vi "posicionador3_2_8_ElBueno_4.vi"() -> ()   [LabVIEW 2015]
uses:
  <vilib>/Instr/_visa.llb/VISA Configure Serial Port (Instr).vi
panel:
  out "Caracterización Terminada":bool
  in  "Puerto Serial del Gaussmetro":refnum<visa-resource-name>="COM5"
  in  "Ruta de archivo de medición":path=path "C:/Users/PIV/Desktop/Enrico/prueba1.txt"
  in  "Dato de entrada para\nobtención de flujo magnético 2":string=":MEASure:FLUX?\n"
  out "Medición de campo magnético \nen Teslas [T]":string
  out "?":string="mm"
  out "?":string="mm"
  in  "Listo Y":bool
  in  "Listo X":bool
  in  "Abajo":bool
  in  "Arriba":bool
  in  "Derecha":bool
  in  "Izquierda":bool
  out "Posiciòn en eje X":i32
  out "Posiciòn en eje Y":i32
  in  "Longitud del imán":i32
  in  "Altura del imán":i32
  in  "Puerto Serial de Arduino":refnum<visa-resource-name>="COM12"
  # "Manual de uso para sistema de monitoreo y control de lecturas de flujo magnético y desplazamiento de posicionador:\n\nSECCI`ÓN DE IDE DE ARDUINO: El archivo se encuentra bajo la x\n\n1.  Los pines para la conexión del driver del motor con el arduino están indicados en el archivo \"motor2.ino\" mediante las variables \"DirPin\", \"StepPin\", \"EnnablePin\" para el motor en X, y \"DirPin2\", \"StepPin2\", \"EnnablePin2\", para el motor en Y. El primer pin refiere a la Dirección; el segundo es el pin para mandarle el tren de pulsos y el tercero para habilitar el motor.\n2.  Para modificar el desplazamiento de 1mm de ambos motores, se deberá modificar el archivo \"motor2.ino\" en la sección después del loop denominada \"void stepMotor\" y \"void Stepmotor2, modificar la variable steps por la cantidad de desplazamiento deseado, tomando en cuenta que steps = 1000 = 1mm de desplazamiento.\n3.  En el apartado \"Puerto Serial de Arduino\" en la parte superior izquierda, indicar el puerto serial del Arduino. Para verificar en què puerto se localiza, dirigirse al menù inicio y escribir \"Administrador de dispositivos\". Seguido de esto se darà click en la opciòn con el mismo nombre y, en la ventaja que emerge, se buscarà el apartado \"Puertos COM y LPT\". El puerto del Arduino lleva por nombre inicial \"Arduino\".\n4.  Para seleccionar el puerto del Gaussmetro, dirigirse como en el paso anterior al Administrador de dispositivos y en el apartado Puerto COM y LPT buscar el nombre \"Prolific USB-to-Serial Comm Port\", y el nombre del puerto se especificarà entre parèntesis. Este nombre de puerto se especificará en el apartado \"Puerto Serial del Gaussmetro\" ubicado debajo del apartado \"Puerto Serial de Arduino\". \n5.  Ingresar la longitud [en mm] del imán.\n6.  Ingresar el alto [en mm] del imán\n7.  Crear un archivo de texto .txt en la computadora (ubicación a elección) para guardar archivos \n8.  En el apartado \"Ruta de archivo de medición\" se deberá introducir la ubicación del archivo creado en el paso anterior. De esta manera, se introducirán las mediciones en este archivo.\n9.  En el apartado \"Dato de entrada para obtención de campo magnético\" se encuentra escrito el comando paara que el Gaussmetro arroje la medición de campo magnético.\n10.  Colocar el imán a caracterizar de forma que la probeta se encuentre del lado superior izquierdo de este. Esto debido a que el movimiento horizontal es hacia la derecha, y el movimiento vertical es hacia abajo.\n11.  Iniciar programa mediante la flecha (con dirección a la derecha) blanca en la parte superior izquierda del panel frontal o Ctrl+R.\n12. Verificar Conexión entre el Arduino y el posicionador. Esto se realiza observando un foco led color naranja en el motor (esto indica que la comunicación serial fue exitosa).\n13.  En caso de estar apagada la luz led naranja del motor, se deberá reiniciar el programa. Esto se consigue oprimiendo el boton \"Listo X\". Al hacer esto, se encenderá el led naranja, y de esta manera se procede a apagar el programa mediante el botón rojo de la parte superior izquierda del panel frontal. Después de realizar esta acciòn, volver a ejecutar el progama oprimiendo la flecha blanca a la izquierda del botón rojo o CTRL+R\n14.  Se deberá iniciar colocando la posición inicial en X (Derecha e Izquierda). Una vez finalizada la posición inicial en X, oprimir el botón \"Listo X\". Al finalizar, deberá parpadear una vez el foco led naranja y se volverá a encender.\n15.  Seguido, se colocará la  posición inicial en Y (Arriba y Abajo). Una vez finalizada la posición inicial en Y, oprimir el botón \"Listo Y\". Al finalizar, deberá parpadear una vez el foco led naranja y se volverá a encender.\n16.  Se comenzará la caracterización deseada.\n\n\nCreado por:\nSebastian A. Reyes Romero\nContacto: rerosa@ier.unam.mx"
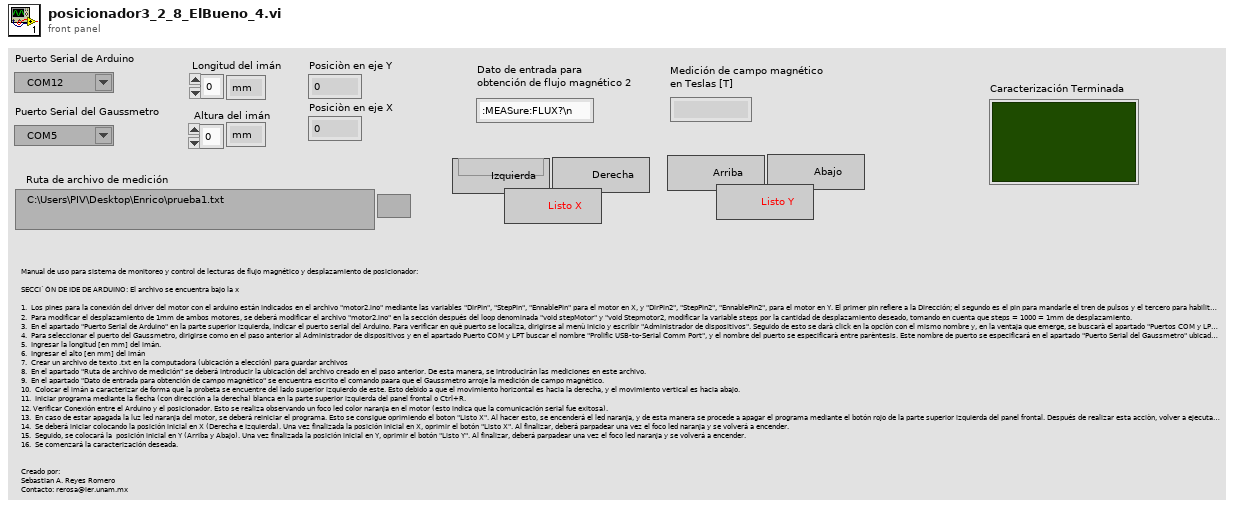
[diagram p1: front panel]
types:
  T1 = enum16{"open", "open or create", "create or replace", "create", "open (read only)"}
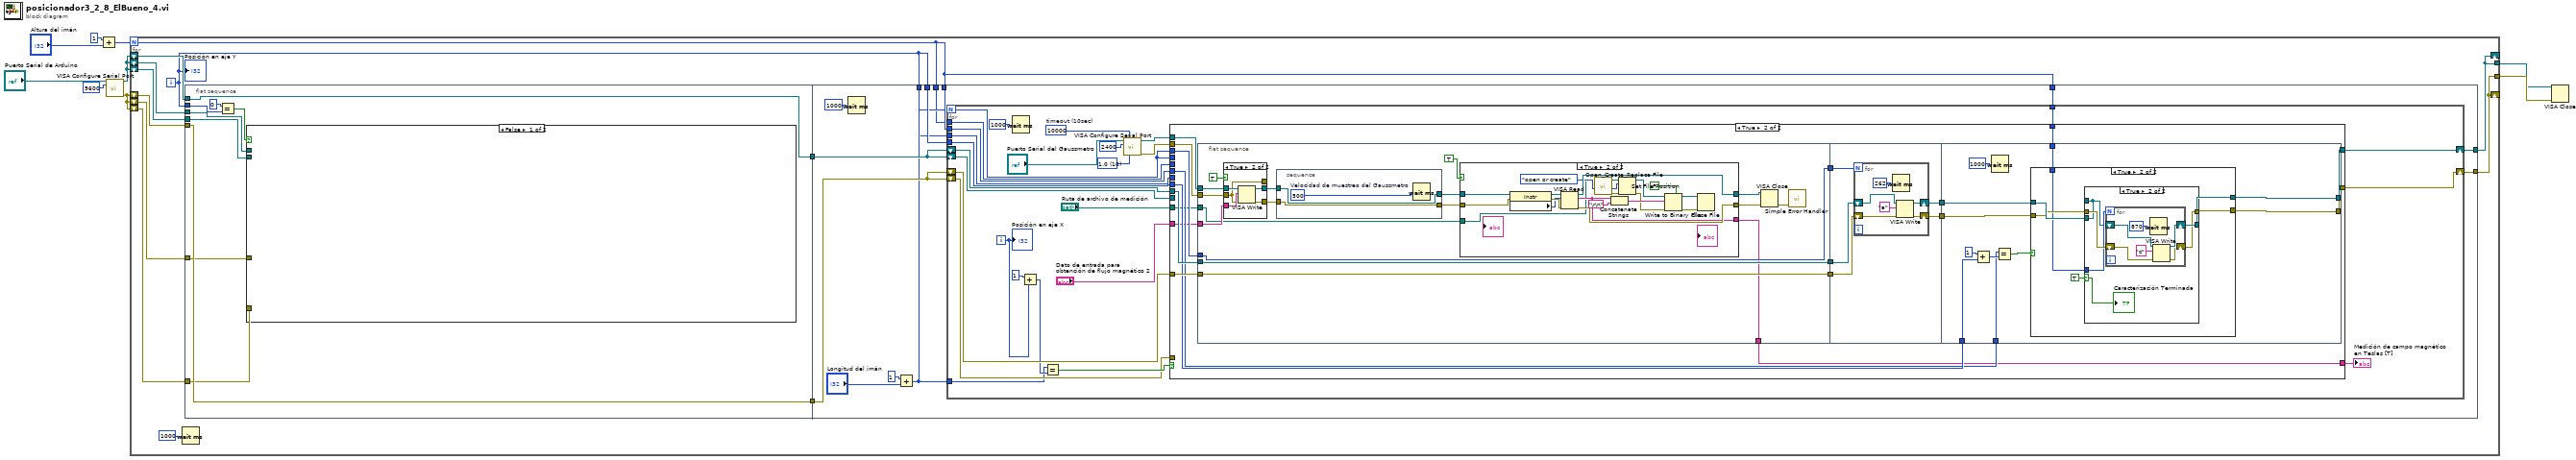
[diagram p0: block diagram]
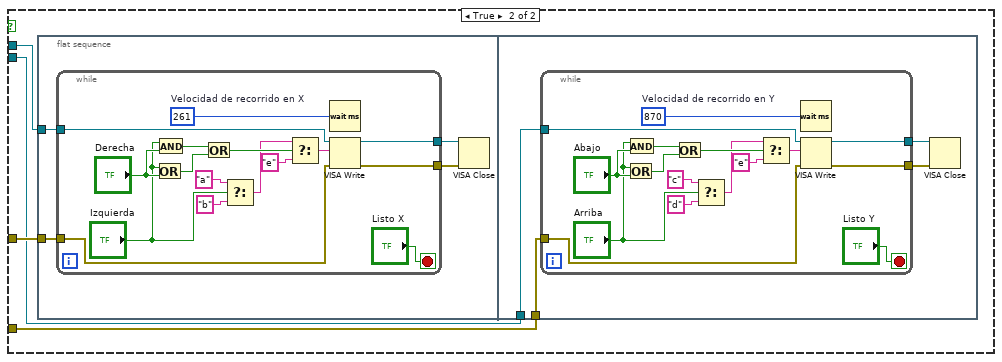
[diagram p2: hidden frame]
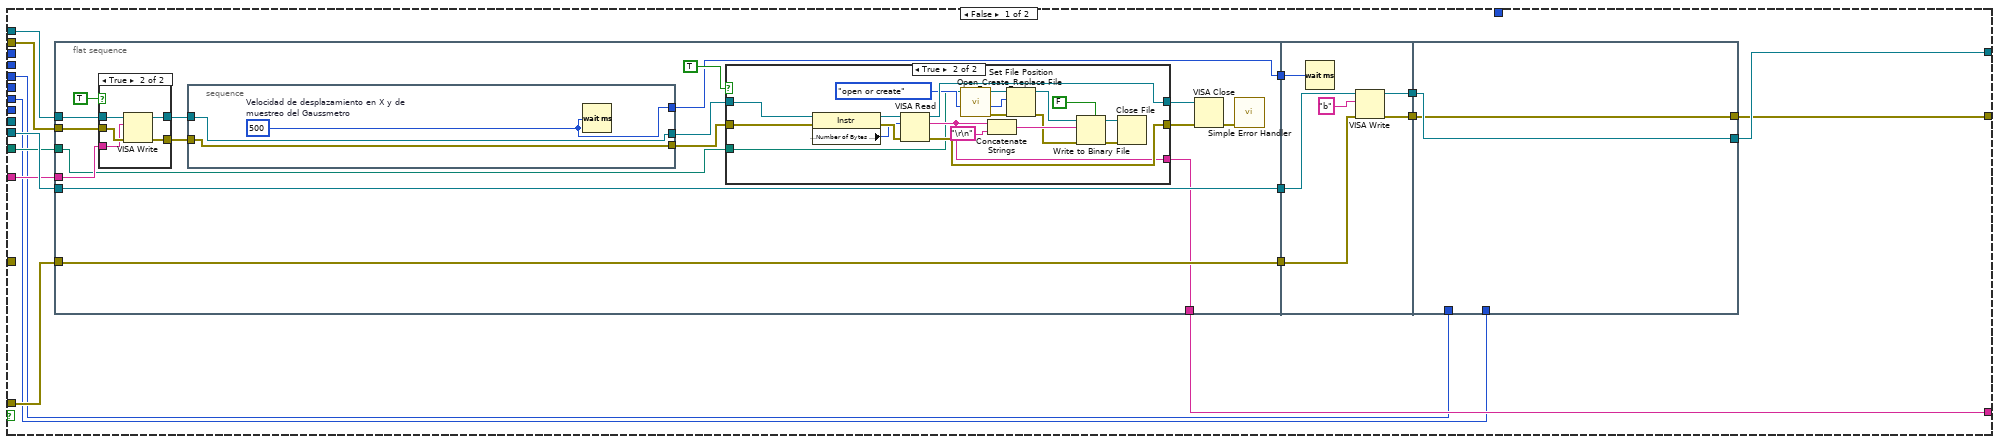
[diagram p3: hidden frame]
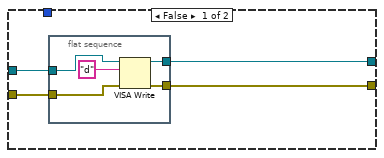
[diagram p8: hidden frame]
diagram:
  n1 = Add(x=1, y="Altura del imán") -> (x+y=w5:i32)
  n2 = call-poly "VISA Configure Serial Port"("VISA resource name"="Puerto Serial de Arduino", "baud rate (9600)"=u32 9600) -> ("VISA resource name out"=w3:refnum<visa-resource-name>, "error out"=w4:errorcluster)  [unwired: 12 in]
  n3 = for {
    N: w5 -> [w10]
    shift-right: [w12] -> _
    shift-right: [w13] -> _
    shift-left: w4 -> [w22]
    shift-left: w3 -> [w18]
    shift-left: w4 -> [w17]
    shift-left: w4 -> [w16]
    shift-left: w3 -> [w14]
    shift-left: w3 -> [w15]
    tunnel: [w13] -> w2
    tunnel: [w12] -> w1
    i -> [w11]
    n4 = Wait (ms)(milliseconds to wait=u32 1000) -> ()  [unwired: 1 out]
    n5 = flat-sequence {
      tunnel: w22 -> [w31]
      tunnel: [w28] -> w20
      tunnel: [w31] -> w19
      tunnel: w18 -> [w27]
      tunnel: w17 -> [w30]
      tunnel: w16 -> [w29]
      tunnel: w15 -> [w28]
      tunnel: w14 -> [w26]
      tunnel: w11 -> [w25]
      tunnel: [w87] -> w13
      tunnel: [w88] -> w12
      tunnel: w11 -> [w84]
      tunnel: w10 -> [w83]
      tunnel: w20 -> [w86]
      tunnel: w19 -> [w85]
      tunnel: w10 -> [w78]
      tunnel: w11 -> [w77]
      tunnel: w10 -> [w76]
      frame #0 {
        n6 = Equal?(x=0, y=w25) -> (x = y?=w23:bool)
        n7 = case shown="False" w23 {
          tunnel: w30 -> [_ w35]
          tunnel: w29 -> [_ w34]
          tunnel: w27 -> [_ w33]
          tunnel: w26 -> [_ w32]
          frame False {
          }
          frame True {
            n8 = flat-sequence {
              tunnel: w32 -> [w39]
              tunnel: w35 -> [w38]
              tunnel: w33 -> [w59]
              tunnel: w34 -> [w58]
              frame #0 {
                n9 = while {
                  tunnel: w39 -> [w46]
                  tunnel: w38 -> [w45]
                  tunnel: [w41] -> w37
                  tunnel: [w40] -> w36
                  stop <- "Listo X" stop-if-true
                  w42 = u32 261  # Velocidad de recorrido en X
                  n10 = Or(x="Izquierda", y="Derecha") -> (x .or. y?=w52:bool)
                  n11 = And(x="Izquierda", y="Derecha") -> (x .and. y?=w54:bool)
                  n12 = Or(x=w54, y=w52) -> (x .or. y?=w51:bool)
                  n13 = Select(t="a", s="Izquierda", f="b") -> (s? t:f=w44:string)
                  n14 = Select(t=w44, s=w51, f="e") -> (s? t:f=w47:string)
                  n15 = Wait (ms)(milliseconds to wait=w42) -> ()  [unwired: 1 out]
                  n16 = VISA Write(VISA resource name=w46, write buffer=w47, error in (no error)=w45) -> (VISA resource name out=w40:refnum<visa-resource-name>, error out=w41:errorcluster)  [unwired: 1 out]
                }
                n17 = VISA Close(VISA resource name=w36, error in (no error)=w37) -> ()  [unwired: 1 out]
              }
              frame #1 {
                n18 = while {
                  tunnel: w59 -> [w66]
                  tunnel: w58 -> [w65]
                  tunnel: [w61] -> w57
                  tunnel: [w60] -> w56
                  stop <- "Listo Y" stop-if-true
                  w62 = u32 870  # Velocidad de recorrido en Y
                  n19 = Or(x="Arriba", y="Abajo") -> (x .or. y?=w73:bool)
                  n20 = And(x="Arriba", y="Abajo") -> (x .and. y?=w74:bool)
                  n21 = Or(x=w74, y=w73) -> (x .or. y?=w72:bool)
                  n22 = Select(t="c", s="Arriba", f="d") -> (s? t:f=w63:string)
                  n23 = Select(t=w63, s=w72, f="e") -> (s? t:f=w67:string)
                  n24 = Wait (ms)(milliseconds to wait=w62) -> ()  [unwired: 1 out]
                  n25 = VISA Write(VISA resource name=w66, write buffer=w67, error in (no error)=w65) -> (VISA resource name out=w60:refnum<visa-resource-name>, error out=w61:errorcluster)  [unwired: 1 out]
                }
                n26 = VISA Close(VISA resource name=w56, error in (no error)=w57) -> ()  [unwired: 1 out]
              }
            }
          }
        }
      }
      frame #1 {
        n27 = Wait (ms)(milliseconds to wait=u32 1000) -> ()  [unwired: 1 out]
        n28 = Add(x=1, y="Longitud del imán") -> (x+y=w80:i32)
        n29 = for {
          N: w80 -> [w109]
          shift-right: [w112] -> w88
          shift-left: w86 -> [w114]
          shift-right: [w111] -> w87
          shift-left: w85 -> [w113]
          shift-left: w86 -> [w110]
          shift-left: w85 -> [w108]
          tunnel: w80 -> [w104]
          tunnel: w84 -> [w103]
          tunnel: w83 -> [w102]
          tunnel: w78 -> [w91]
          tunnel: w77 -> [w90]
          tunnel: w76 -> [w89]
          i -> [w107]
          w94 = u16 10 items=["1.0"=10, "1.5"=15, "2.0"=20] ("stop bits (10: 1 bit)")
          w97 = u32 10000  # timeout (10sec)
          n30 = Wait (ms)(milliseconds to wait=u32 1000) -> ()  [unwired: 1 out]
          n31 = Add(x=1, y=w107) -> (x+y=w105:i32)
          n32 = Equal?(x=w104, y=w105) -> (x = y?=w115:bool)
          n33 = call-poly "VISA Configure Serial Port"("VISA resource name"="Puerto Serial del Gaussmetro", "timeout (10sec)"=w97, "baud rate (9600)"=u32 2400, "stop bits (10: 1 bit)"=w94) -> ("VISA resource name out"=w93:refnum<visa-resource-name>, "error out"=w92:errorcluster)  [unwired: 5 in, 5 out]
          n34 = case shown="True" w115 {
            tunnel: w114 -> [_ w206]
            tunnel: w113 -> [_ w205]
            tunnel: [w129 w204] -> w112
            tunnel: [w128 w203] -> w111
            tunnel: w109 -> [_ w202]
            tunnel: w110 -> [w131 _]
            tunnel: w108 -> [w130 _]
            tunnel: w109 -> [_ _]
            tunnel: w103 -> [_ w199]
            tunnel: w102 -> [_ w198]
            tunnel: [w124 w194] -> w100
            tunnel: "Dato de entrada para\nobtención de flujo magnético 2" -> [w123 w193]
            tunnel: "Ruta de archivo de medición" -> [w122 w192]
            tunnel: w93 -> [w121 w191]
            tunnel: w92 -> [w120 w190]
            tunnel: w91 -> [w117 _]
            tunnel: w90 -> [w116 _]
            tunnel: w89 -> [_ w189]
            frame False {
              n35 = flat-sequence {
                tunnel: w130 -> [w147]
                tunnel: w131 -> [w148]
                tunnel: [w148] -> w127
                tunnel: [w147] -> w126
                tunnel: [w137] -> w125
                tunnel: [w136] -> w124
                tunnel: w123 -> [w135]
                tunnel: w122 -> [w134]
                tunnel: w121 -> [w133]
                tunnel: w120 -> [w132]
                tunnel: w127 -> [w186]
                tunnel: w126 -> [w185]
                tunnel: w125 -> [w181]
                tunnel: [w184] -> w119
                tunnel: [w183] -> w118
                tunnel: [w187] -> w128
                tunnel: [w188] -> w129
                tunnel: w119 -> [w188]
                tunnel: w118 -> [w187]
                tunnel: w117 -> [_]
                tunnel: w116 -> [_]
                frame #0 {
                  n36 = case shown="True" TRUE ("write") {
                    tunnel: [w153 w158] -> w141
                    tunnel: w133 -> [w152 w157]
                    tunnel: w132 -> [w153 w156]
                    tunnel: [w152 w155] -> w139
                    tunnel: w135 -> [_ w154]
                    frame False {
                    }
                    frame True {
                      n37 = VISA Write(VISA resource name=w157, write buffer=w154, error in (no error)=w156) -> (VISA resource name out=w155:refnum<visa-resource-name>, error out=w158:errorcluster)  [unwired: 1 out]
                    }
                  }
                  n38 = stacked-sequence {
                    tunnel: w141 -> [w151]
                    tunnel: [w151] -> w140
                    tunnel: w139 -> [w150]
                    tunnel: [w150] -> w138
                    tunnel: [w149] -> w137
                    frame #0 {
                      w149 = u32 500  # Velocidad de desplazamiento en X y de muestreo del Gaussmetro
                      n39 = Wait (ms)(milliseconds to wait=w149) -> ()  [unwired: 1 out]
                    }
                  }
                  n40 = case shown="True" TRUE ("read") {
                    tunnel: w140 -> [w160 w177]
                    tunnel: [w160 w174] -> w145
                    tunnel: [w159 w180] -> w144
                    tunnel: w138 -> [w159 w179]
                    tunnel: [_ w162] -> w136
                    tunnel: w134 -> [_ w161]
                    frame False {
                    }
                    frame True {
                      n41 = property class="Instr"(reference=w179, error in=w177) -> (reference out=w178:refnum<visa-resource-name>, error out=w176:errorcluster, "Serial Settings:Number of Bytes at Serial Port"=w175:u32)
                      n42 = VISA Read(VISA resource name=w178, byte count=w175, error in (no error)=w176) -> (VISA resource name out=w180:refnum<visa-resource-name>, read buffer=w162:string, error out=w174:errorcluster)  [unwired: 1 out]
                      n43 = call <vilib>:"Open_Create_Replace File.vi"("function (open:0)"=T1."open or create", "file path"=w161) -> ("error out"=w172:errorcluster, "file size (bytes)"=w170:i32, "refnum"=w171:refnum<file>)  [unwired: 6 in, 1 out]
                      n44 = Concatenate Strings(w162, "\r\n") -> (w166:string)
                      n45 = Set File Position(offset (in bytes) (0)=w170, refnum=w171, error in=w172) -> (refnum out=w165:refnum<file>, error out=w164:errorcluster)  [unwired: 1 in]
                      n46 = Write to Binary File(file (use dialog)=w165, data=w166, error in=w164, 5:FALSE ("prepend array or string size? (T)")) -> (refnum out=w168:refnum<file>, error out=w169:errorcluster)  [unwired: 2 in, 1 out]
                      n47 = Close File(refnum=w168, error in=w169) -> ()  [unwired: 2 out]
                    }
                  }
                  n48 = VISA Close(VISA resource name=w144, error in (no error)=w145) -> (error out=w143:errorcluster)
                  n49 = call <vilib>:"Simple Error Handler.vi"("error in (no error)"=w143) -> ()  [unwired: 1 in, 8 out]
                }
                frame #1 {
                  n50 = Wait (ms)(milliseconds to wait=w181) -> ()  [unwired: 1 out]
                  n51 = VISA Write(VISA resource name=w186, write buffer="b", error in (no error)=w185) -> (VISA resource name out=w184:refnum<visa-resource-name>, error out=w183:errorcluster)  [unwired: 1 out]
                }
                frame #2 {
                }
              }
            }
            frame True {
              n52 = flat-sequence {
                tunnel: w202 -> [w221]
                tunnel: w205 -> [w222]
                tunnel: w206 -> [w223]
                tunnel: [w223] -> w197
                tunnel: [w222] -> w196
                tunnel: [w221] -> w195
                tunnel: [w211] -> w194
                tunnel: w193 -> [w210]
                tunnel: w192 -> [w209]
                tunnel: w191 -> [w208]
                tunnel: w190 -> [w207]
                tunnel: [w258] -> w201
                tunnel: [w257] -> w200
                tunnel: w197 -> [w260]
                tunnel: w196 -> [w259]
                tunnel: w195 -> [w256]
                tunnel: [w276] -> w203
                tunnel: [w277] -> w204
                tunnel: w198 -> [w270]
                tunnel: w199 -> [w273]
                tunnel: w200 -> [w274]
                tunnel: w201 -> [w275]
                tunnel: w189 -> [w267]
                frame #0 {
                  n53 = case shown="True" TRUE ("write 2") {
                    tunnel: [w227 w233] -> w215
                    tunnel: w208 -> [w228 w232]
                    tunnel: [w227 w229] -> _
                    tunnel: [w228 w231] -> w213
                    tunnel: w210 -> [_ w230]
                    tunnel: w207 -> [w227 w229]
                    frame False {
                    }
                    frame True {
                      n54 = VISA Write(VISA resource name=w232, write buffer=w230, error in (no error)=w229) -> (VISA resource name out=w231:refnum<visa-resource-name>, error out=w233:errorcluster)  [unwired: 1 out]
                    }
                  }
                  n55 = stacked-sequence {
                    tunnel: w215 -> [w226]
                    tunnel: [w226] -> w214
                    tunnel: w213 -> [w225]
                    tunnel: [w225] -> w212
                    frame #0 {
                      w224 = u32 500  # Velocidad de muestreo del Gaussmetro
                      n56 = Wait (ms)(milliseconds to wait=w224) -> ()  [unwired: 1 out]
                    }
                  }
                  n57 = case shown="True" TRUE ("read 2") {
                    tunnel: w214 -> [w235 w252]
                    tunnel: [w235 w249] -> w219
                    tunnel: [w234 w255] -> w218
                    tunnel: w212 -> [w234 w254]
                    tunnel: [_ w237] -> w211
                    tunnel: w209 -> [_ w236]
                    frame False {
                    }
                    frame True {
                      n58 = property class="Instr"(reference=w254, error in=w252) -> (reference out=w253:refnum<visa-resource-name>, error out=w251:errorcluster, "Serial Settings:Number of Bytes at Serial Port"=w250:u32)
                      n59 = VISA Read(VISA resource name=w253, byte count=w250, error in (no error)=w251) -> (VISA resource name out=w255:refnum<visa-resource-name>, read buffer=w237:string, error out=w249:errorcluster)  [unwired: 1 out]
                      n60 = call <vilib>:"Open_Create_Replace File.vi"("function (open:0)"=T1."open or create", "file path"=w236) -> ("error out"=w247:errorcluster, "file size (bytes)"=w245:i32, "refnum"=w246:refnum<file>)  [unwired: 6 in, 1 out]
                      n61 = Concatenate Strings(w237, "\r\n") -> (w241:string)
                      n62 = Set File Position(offset (in bytes) (0)=w245, refnum=w246, error in=w247) -> (refnum out=w240:refnum<file>, error out=w239:errorcluster)  [unwired: 1 in]
                      n63 = Write to Binary File(file (use dialog)=w240, data=w241, error in=w239, 5:FALSE ("prepend array or string size? (T)")) -> (refnum out=w243:refnum<file>, error out=w244:errorcluster)  [unwired: 2 in, 1 out]
                      n64 = Close File(refnum=w243, error in=w244) -> ()  [unwired: 2 out]
                    }
                  }
                  n65 = VISA Close(VISA resource name=w218, error in (no error)=w219) -> (error out=w217:errorcluster)
                  n66 = call <vilib>:"Simple Error Handler.vi"("error in (no error)"=w217) -> ()  [unwired: 1 in, 8 out]
                }
                frame #1 {
                  n67 = for {
                    N: w256 -> [_]
                    shift-right: [w264] -> w258
                    shift-left: w260 -> [w266]
                    shift-right: [w263] -> w257
                    shift-left: w259 -> [w265]
                    n68 = Wait (ms)(milliseconds to wait=u32 262) -> ()  [unwired: 1 out]
                    n69 = VISA Write(VISA resource name=w266, write buffer="a", error in (no error)=w265) -> (VISA resource name out=w264:refnum<visa-resource-name>, error out=w263:errorcluster)  [unwired: 1 out]
                  }
                }
                frame #2 {
                  n70 = Add(x=1, y=w273) -> (x+y=w271:i32)
                  n71 = Wait (ms)(milliseconds to wait=u32 1000) -> ()  [unwired: 1 out]
                  n72 = Equal?(x=w270, y=w271) -> (x = y?=w269:bool)
                  n73 = case shown="True" w269 {
                    tunnel: w275 -> [w281 w292]
                    tunnel: [w280 w290] -> w277
                    tunnel: w274 -> [w279 w291]
                    tunnel: [w278 w289] -> w276
                    tunnel: w267 -> [_ w288]
                    frame False {
                      n74 = flat-sequence {
                        tunnel: [w285] -> w278
                        tunnel: [w286] -> w280
                        tunnel: w279 -> [w283]
                        tunnel: w281 -> [w284]
                        frame #0 {
                          n75 = VISA Write(VISA resource name=w284, write buffer="d", error in (no error)=w283) -> (VISA resource name out=w286:refnum<visa-resource-name>, error out=w285:errorcluster)  [unwired: 1 out]
                        }
                      }
                    }
                    frame True {
                      n76 = case shown="True" TRUE {
                        selector: TRUE -> [_ w295]
                        tunnel: [w293 w296] -> _
                        tunnel: w291 -> [w294 w300]
                        tunnel: [w293 w299] -> w290
                        tunnel: [w294 w298] -> w289
                        tunnel: w288 -> [_ w297]
                        tunnel: w292 -> [w293 w296]
                        frame False {
                        }
                        frame True {
                          n77 = for {
                            N: w297 -> [_]
                            shift-right: [w304] -> w299
                            shift-left: w296 -> [w306]
                            shift-right: [w303] -> w298
                            shift-left: w300 -> [w305]
                            n78 = Wait (ms)(milliseconds to wait=u32 870) -> ()  [unwired: 1 out]
                            n79 = VISA Write(VISA resource name=w306, write buffer="c", error in (no error)=w305) -> (VISA resource name out=w304:refnum<visa-resource-name>, error out=w303:errorcluster)  [unwired: 1 out]
                          }
                          "Caracterización Terminada" <- w295
                        }
                      }
                    }
                  }
                }
              }
            }
          }
          "Medición de campo magnético \nen Teslas [T]" <- w100
          "Posiciòn en eje X" <- w107
        }
      }
    }
    "Posiciòn en eje Y" <- w11
  }
  n80 = VISA Close(VISA resource name=w1, error in (no error)=w2) -> ()  [unwired: 1 out]
